vi "create.vi"(8 "error in":errorcluster, 9 "handler properties":T1={"max url size"=8000, "max header"=8000, "timeout ms"=5000, "max data size"=104857600}, 10 "connection handler pool size":i32=10, 11 "port":u16=80) -> (0 "error out":errorcluster, 3 "Basic HTTP server out":refnum<class "Basic HTTP server.lvclass">)   [LabVIEW 2013, in "Basic HTTP server.lvclass"]
uses:
  Basic HTTP server.lvclass
  http server properties.ctl
  Basic HTTP server.lvclass/Basic HTTP server.ctl
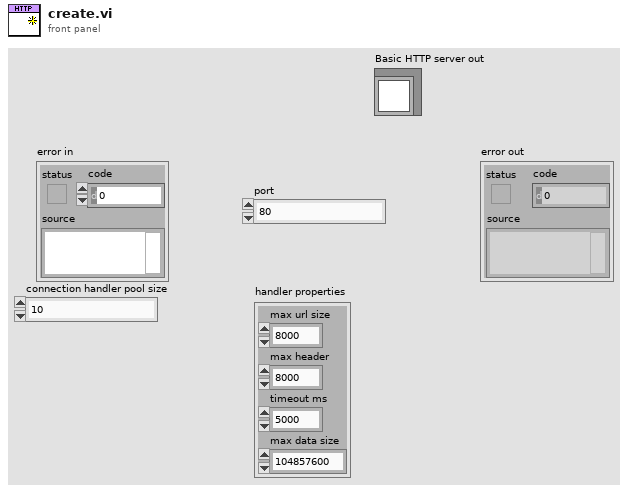
[diagram p1: front panel]
types:
  T1 = typedef "Basic HTTP server.lvclass/http server properties.ctl" = cluster{"max url size":i32, "max header":i32, "timeout ms":i32, "max data size":i32}
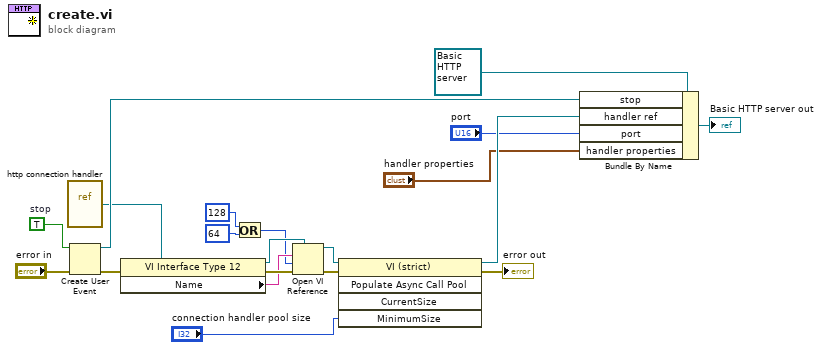
[diagram p0: block diagram]
diagram:
  w19 = TRUE  # stop
  n1 = vi-ref "http connection handler.vi"() -> (w1:refnum<vi>)
  n2 = Create User Event(user event datatype=w19, error in="error in") -> (user event=w17:refnum<user-event>, error out=w6:errorcluster)
  n3 = property class="VI Interface Type 12"(reference=w1, error in=w6) -> (reference out=w12:refnum<vi>, error out=w15:errorcluster, "Name"=w13:string)
  n4 = Or(x=128 ("options"), y=64 ("options")) -> (x .or. y?=w11:i32)
  n5 = Open VI Reference(type specifier VI Refnum (for type only)=w12, vi path=w13, options=w11, error in (no error)=w15) -> (vi reference=w9:refnum<vi>, error out=w14:errorcluster)  [unwired: 2 in]
  n6 = invoke class="VI (strict)" method="Populate Async Call Pool"(reference=w9, error in=w14, "MinimumSize"="connection handler pool size") -> (reference out=w4:refnum<vi>, error out=→"error out":errorcluster)  [unwired: 2 in, 3 out]
  n7 = Bundle By Name(cluster=refnum<class "Basic HTTP server.lvclass"> refnum ("Basic HTTP server in"), "stop"=w17, "handler ref"=w4, "port"="port", "handler properties"="handler properties") -> (→"Basic HTTP server out":refnum<class "Basic HTTP server.lvclass">)
